vi "solar_msg Qs Shutdown.vi"(8 "error in (no error)":errorcluster, 9 "sec Timeout (60)":u32=60, 11 "Queue Names":string[](array[string])) -> (0 "error out":errorcluster, 1 "Timed Out?":bool)   [LabVIEW 2018]
doc: "This VI waits for all <b>Queues</b> to shutdown. The <b>sec Timeout</b> specifies the time to wait for all queues to become invalid."
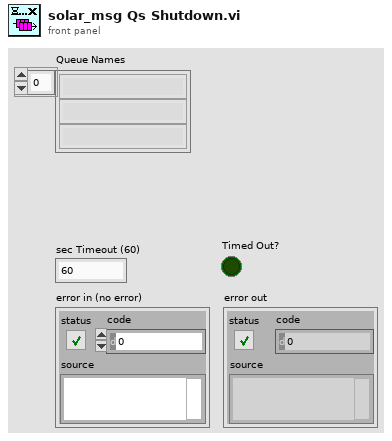
[diagram p1: front panel]
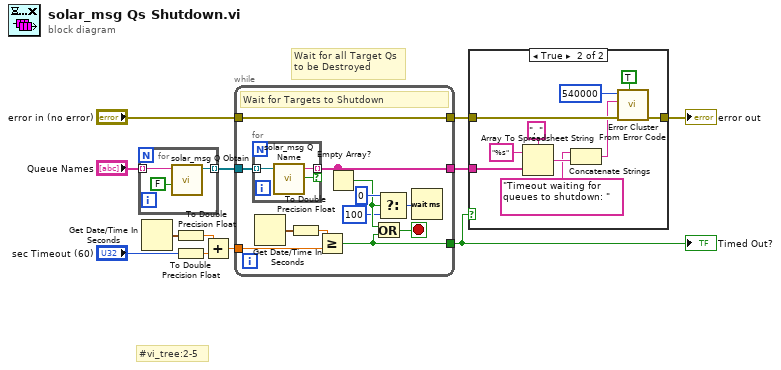
[diagram p0: block diagram]
diagram:
  # "#vi_tree:2-5"
  # "Wait for all Target Qs\nto be Destroyed"
  n1 = for {
    tunnel: "Queue Names" -> [w15] mode=indexing
    tunnel: [w13] -> w1 mode=indexing
    n2 = call "solar_msg Q Obtain.vi"("Create If Not Found? (T)"=FALSE, "Queue Name (unnamed)"=w15) -> ("Queue"=w13:refnum<queue>)  [unwired: 7 in, 2 out]
  }
  n3 = Get Date/Time In Seconds() -> (seconds since 1Jan1904=w12:timestamp)
  n4 = To Double Precision Float(number=w12) -> (double precision float=w11:dbl)
  n5 = To Double Precision Float(number="sec Timeout (60)") -> (double precision float=w10:dbl)
  n6 = Add(x=w11, y=w10) -> (x+y=w9:dbl)
  n7 = while {
    tunnel: w1 -> [w19]
    tunnel: w9 -> [w26]
    tunnel: [w21] -> w8
    tunnel: "error in (no error)" -> [w21]
    tunnel: [w20] -> w3
    tunnel: [w18] -> w4
    stop <- w24 stop-if-true
    # "Wait for Targets to Shutdown"
    n8 = for {
      tunnel: w19 -> [w30] mode=indexing
      tunnel: [w29] -> w18 mode=indexing if=w28
      n9 = call "solar_msg Q Name.vi"("Queue"=w30) -> ("Valid Queue?"=w28:bool, "Queue Name"=w29:string)  [unwired: 7 in]
    }
    n10 = Get Date/Time In Seconds() -> (seconds since 1Jan1904=w27:timestamp)
    n11 = To Double Precision Float(number=w27) -> (double precision float=w25:dbl)
    n12 = Greater Or Equal?(x=w25, y=w26) -> (x >= y?=w20:bool)
    n13 = Empty Array?(array=w18) -> (empty?=w17:bool)
    n14 = Or(x=w17, y=w20) -> (x .or. y?=w24:bool)
    n15 = Select(t=u32 0, s=w17, f=u32 100 ("msWait")) -> (s? t:f=w22:u32)
    n16 = Wait (ms)(milliseconds to wait=w22) -> ()  [unwired: 1 out]
  }
  "Timed Out?" <- w3
  n17 = case shown="True" w3 {
    tunnel: w8 -> [w31 w41]
    tunnel: [w31 w40] -> w6
    tunnel: w4 -> [_ w37]
    frame False {
      # "All targets shutdown"
    }
    frame True {
      n18 = Array To Spreadsheet String(delimiter (Tab)=", ", array=w37, 3:"%s" ("format string")) -> (spreadsheet string=w34:string)
      n19 = Concatenate Strings("Timeout waiting for queues to shutdown: " ("source"), w34) -> (w32:string)
      n20 = call <vilib>:"Error Cluster From Error Code.vi"("show call chain? (False)"=TRUE, "error in (no error)"=w41, "error message (\"\")"=w32, "error code (0)"=540000 ("code")) -> ("error out"=w40:errorcluster)  [unwired: 5 in]
    }
  }
  "error out" <- w6
